vi "tangente normalise.vi"(10 "a":dbl, 11 "b":dbl) -> (3 "angle":dbl)   [LabVIEW 2018]
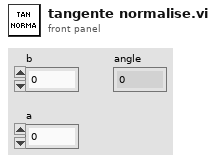
[diagram p1: front panel]
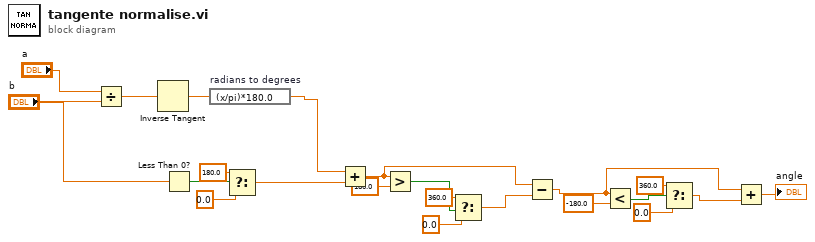
[diagram p0: block diagram]
diagram:
  n1 = Divide(x="a", y="b") -> (x/y=w22:dbl)
  n2 = Inverse Tangent(1:w22) -> (0:w21:dbl)
  n3 = Less Than 0?(x="b") -> (x < 0?=w19:bool)
  n4 = expression code="(x/pi)*180.0" "radians to degrees"(w21) -> (w14:dbl)
  n5 = Select(t=180.0, s=w19, f=0.0) -> (s? t:f=w18:dbl)
  n6 = Add(x=w14, y=w18) -> (x+y=w13:dbl)
  n7 = Greater?(x=w13, y=180.0) -> (0:w10:bool)
  n8 = Select(t=360.0, s=w10, f=0.0) -> (s? t:f=w9:dbl)
  n9 = Subtract(x=w13, y=w9) -> (x-y=w2:dbl)
  n10 = Less?(x=w2, y=-180.0) -> (x < y?=w6:bool)
  n11 = Select(t=360.0, s=w6, f=0.0) -> (s? t:f=w3:dbl)
  n12 = Add(x=w2, y=w3) -> (x+y=→"angle":dbl)
